vi "MRU_GetMRULIst.vi"(8 "error in (no error)":errorcluster, 11 "reference in":refnum<class "MRU.lvclass">) -> (0 "error out":errorcluster, 3 "reference out":refnum<class "MRU.lvclass">)   [LabVIEW 2014, in "MRU.lvclass"]
doc: "Populates the ComboBox with the values in the MRU list. Uses the cached ComboBox reference passed into the constructor."
uses:
  MRU.lvclass
  <vilib>/Utility/config.llb/Read Key (String).vi
  <vilib>/Utility/config.llb/NI_LVConfig.lvlib
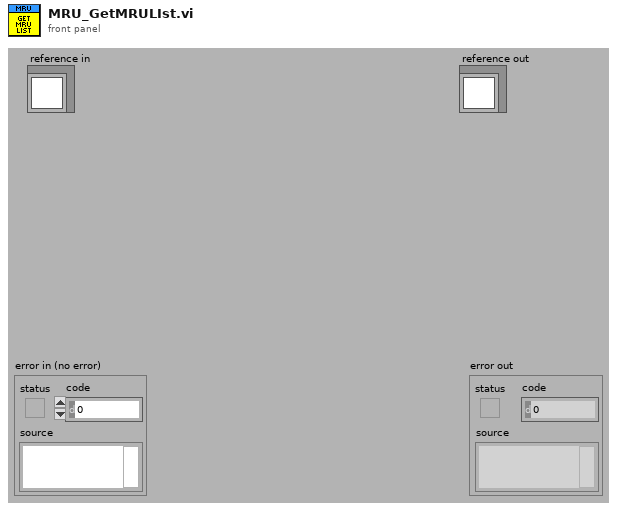
[diagram p1: front panel]
types:
  T1 = typedef "MRU.lvclass/ObjectAttributes.ctl" = cluster{"MRU INI file":path, "MRU Section Name":string, "CmbBox Refnum":refnum<vi>, "Number to remember":i32}
  T2 = typedef "NI_LVConfig.lvlib/Config Data RefNum.ctl" = refnum<k1>
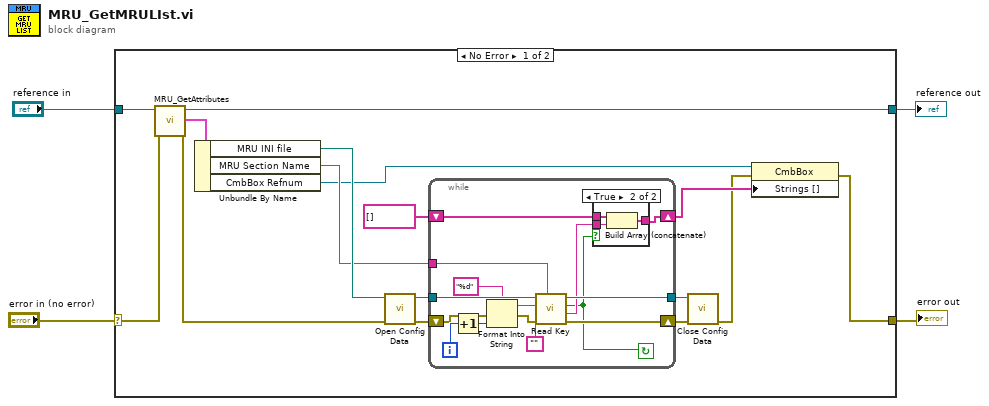
[diagram p0: block diagram]
diagram:
  n1 = case shown="No Error" "error in (no error)" {
    selector: "error in (no error)" -> [w20 w41]
    tunnel: [w6 w41] -> w3
    tunnel: [w18 w40] -> w1
    tunnel: "reference in" -> [w19 w40]
    frame No Error {
      n2 = call "MRU_GetAttributes.vi"("error in (no error)"=w20, "reference in"=w19) -> ("error out"=w7:errorcluster, "Data"=w5:T1, "reference out"=w18:refnum<class "MRU.lvclass">)  [unwired: 6 in, 1 out]
      n3 = Unbundle By Name(w5) -> ("MRU INI file"=w12:path, "MRU Section Name"=w11:string, "CmbBox Refnum"=w10:refnum<vi>)
      n4 = call <vilib>:"Open Config Data.vi"("error in (no error)"=w7, "configuration file path"=w12) -> ("error out"=w14:errorcluster, "refnum"=w16:T2)  [unwired: 7 in, 1 out]
      n5 = while {
        tunnel: w16 -> [w34]
        tunnel: [w33] -> w17
        shift-right: [w35] -> w15
        shift-left: w14 -> [w28]
        tunnel: w11 -> [w32]
        shift-right: [w23] -> w9
        shift-left: string[] [] -> [w24]
        i -> [w30]
        stop <- w22 continue-if-true
        n6 = Increment(x=w30) -> (x+1=w21:i32)
        n7 = Format Into String(format string="%d", error in=w28, w21) -> (resulting string=w29:string, error out=w27:errorcluster)  [unwired: 1 in]
        n8 = call-poly <vilib>:"Read Key.vi"("section"=w32, "error in (no error)"=w27, "default value"="", "key"=w29, "refnum"=w34) -> ("error out"=w35:errorcluster, "value"=w25:string, "found?"=w22:bool, "refnum out"=w33:T2)  [unwired: 1 in, 2 out]
        n9 = case shown="True" w22 {
          tunnel: w25 -> [_ w39]
          tunnel: w24 -> [w36 w38]
          tunnel: [w36 w37] -> w23
          frame False {
          }
          frame True {
            n10 = Build Array (concatenate)(w38, w39) -> (w37:string[])
          }
        }
      }
      n11 = call <vilib>:"Close Config Data.vi"("error in (no error)"=w15, "refnum"=w17) -> ("error out"=w8:errorcluster)  [unwired: 1 in, 8 out]
      n12 = property class="CmbBox"(reference=w10, error in=w8, "Strings []"=w9) -> (error out=w6:errorcluster)  [unwired: 1 out]
    }
    frame Error {
    }
  }
  "error out" <- w3
  "reference out" <- w1
